vi "Read RxTx.lvclass.vi"(8 "error in (no error)":errorcluster, 11 "SPARC4_GUI in":refnum<class "SPARC4_GUI.lvclass">) -> (0 "error out":errorcluster, 2 "RxTx.lvclass":refnum<class "RxTx.lvclass">, 3 "SPARC4_GUI out":refnum<class "SPARC4_GUI.lvclass">)   [LabVIEW 2018, in "SPARC4_GUI.lvclass"]
uses:
  SPARC4_GUI.lvclass
  RxTx/RxTx.lvclass
  SPARC4_GUI.lvclass/SPARC4_GUI.ctl
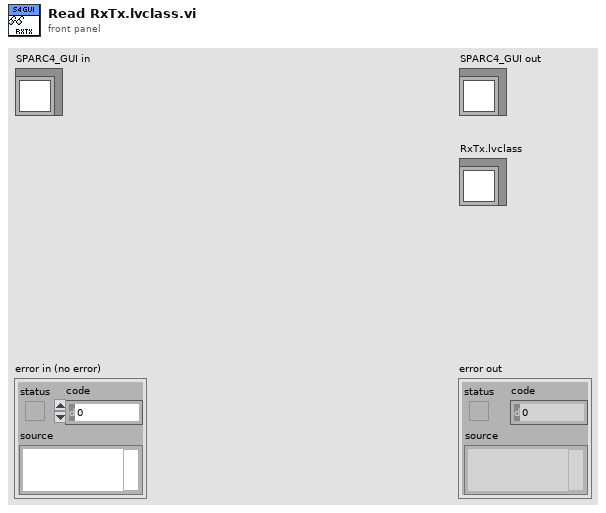
[diagram p1: front panel]
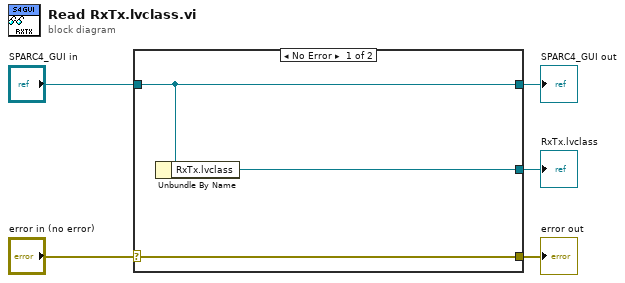
[diagram p0: block diagram]
diagram:
  n1 = case shown="No Error" "error in (no error)" {
    selector: "error in (no error)" -> [w8 w9]
    tunnel: [w8 w9] -> w4
    tunnel: [w7 w10] -> w2
    tunnel: "SPARC4_GUI in" -> [w7 w10]
    tunnel: [w6 _] -> w1
    frame No Error {
      n2 = Unbundle By Name(w7) -> ("RxTx.lvclass"=w6:refnum<class "RxTx.lvclass">)
    }
    frame Error {
    }
  }
  "error out" <- w4
  "SPARC4_GUI out" <- w2
  "RxTx.lvclass" <- w1
